vi "ScaleGetObjId.vi"(4 "error IO":errorcluster, 5 "channel name":string, 6 "group name":string, 7 "tdms file":refnum<k34>) -> (0 "error out":errorcluster, 1 "dll path":path, 2 "objId":u32, 3 "fileId":u32)   [LabVIEW 2017]
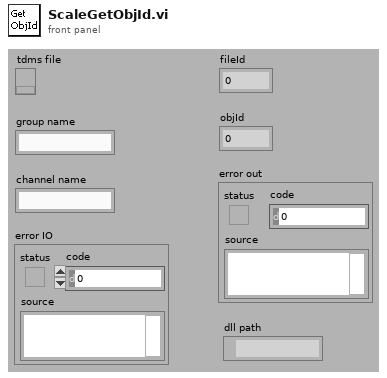
[diagram p1: front panel]
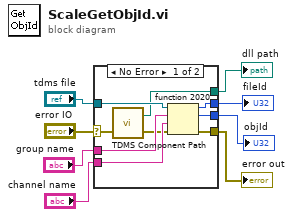
[diagram p0: block diagram]
diagram:
  n1 = case shown="No Error" "error IO" {
    selector: "error IO" -> [w16 w18]
    tunnel: [w13 w18] -> w8
    tunnel: "channel name" -> [w14 _]
    tunnel: "group name" -> [w15 _]
    tunnel: "tdms file" -> [w17 _]
    tunnel: [w12 _] -> w3
    tunnel: [w11 _] -> w2
    tunnel: [w9 _] -> w1
    frame No Error {
      n2 = call <vilib>:"TDMS Component Path.vi"("error in (no error)"=w16) -> ("error out"=w10:errorcluster, "appended path"=w9:path)  [unwired: 1 out]
      n3 = fn#2020(4:w10, 5:w14, 6:w15, 7:w17) -> (0:w13:errorcluster, 2:w11:u64, 3:w12:u64)
    }
    frame Error {
    }
  }
  "error out" <- w8
  "objId" <- w2
  "fileId" <- w3
  "dll path" <- w1
